vi "Select_Alternative_channel.vi"(4 "Filetype":string, 5 "All Tabulated Channels":string[](array[string]), 6 "Reading Filename":path, 7 "Start of data (bytes)":i32, 8 "Template Channel Name":string, 9 "Data string":string, 10 "Previous Channels used":string[](array[string])) -> (0 "Chosen Channel":string, 3 "Selected Index":i32)   [LabVIEW 2016]
uses:
  Results_plotter_Global.vi
panel:
  in  "Cancel Button":bool
  out "Channel Values":dbl[](graph)
  out "Channel Values":string[](array[string])
  out "Message":string
  in  "Boolean":bool
  in  "Select channel to be used":u16(ring) items=["No Suitable Channel Found", "No Suitable Channel Found, Don't Prompt again", "MyFirstName:MySecondName:Frequency (Hz)", "MyFirstName:MySecondName:Boost", "MyFirstName:MySecondName:Phase", "Port::", "L (ft)::", "Tube::", "Trans DeadL (in)::", "Pitot DeadL (in)::", "pold^2/pref^2::", "pnew^2/pref^2::", "pref^2::", "pold^2::", "pnew^2::", "User Comments::", "Pref Mean (V)::", "Pold Mean (V)::", "Pnew Mean (V)::", "Pref Timescale Estimate (s)::", "Pold Timescale Estimate (s)::", "Pnew Timescale Estimate (s)::", "Date of Measurement::", "Time Measurement Commenced::", "Seconds since 1st Jan::", "Measuring Instrument Type::", "Run Messages::", "Av Analogue Sampling Rate::", "No of Analogue Samples::", "No Of Measurement Blocks::", "Flow Measurement Time::", "Prog Post Process Mode::", "Acquisition PlugIn Used::", "Initial PlugIns Used::", "Per Block PlugIns Used::", "Raw Data Filename::", "Current:File:", "Current:File:1st Folder level", "Current:File:2nd Folder level", "Current:File:3rd Folder level", "Current:File:4th Folder level", "Current:File:Number"]
  # "#ToDo- add filter to make it easier to find channels!"
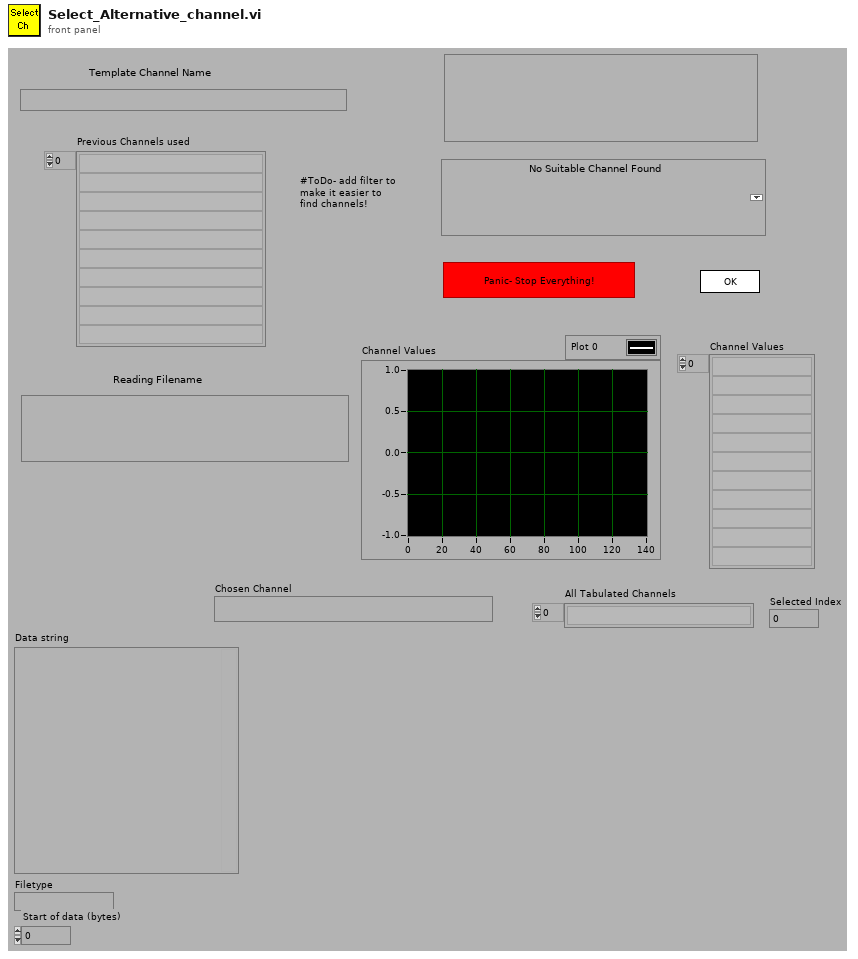
[diagram p1: front panel]
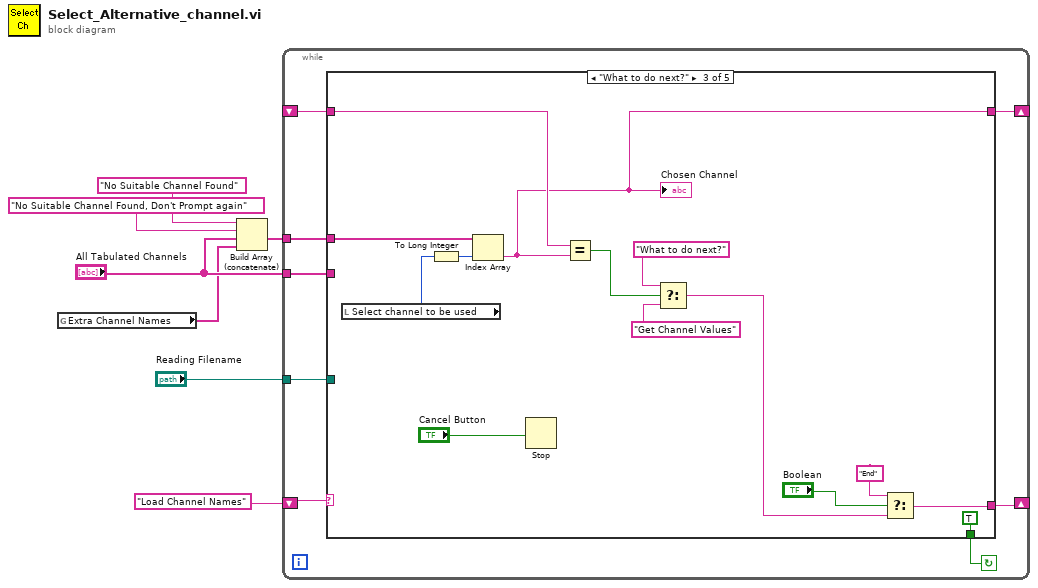
[diagram p0: block diagram]
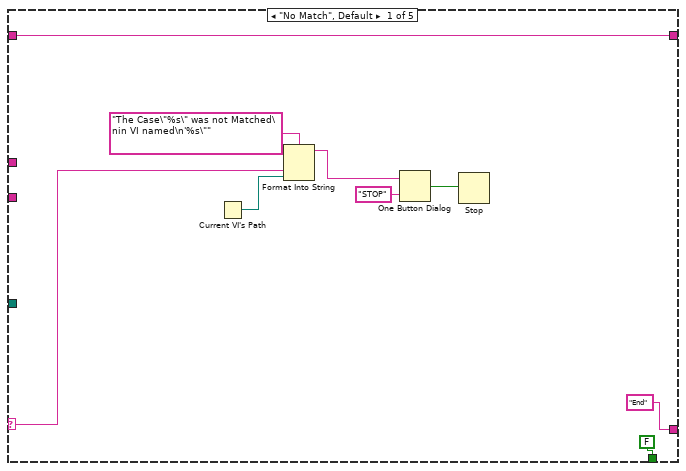
[diagram p2: hidden frame]
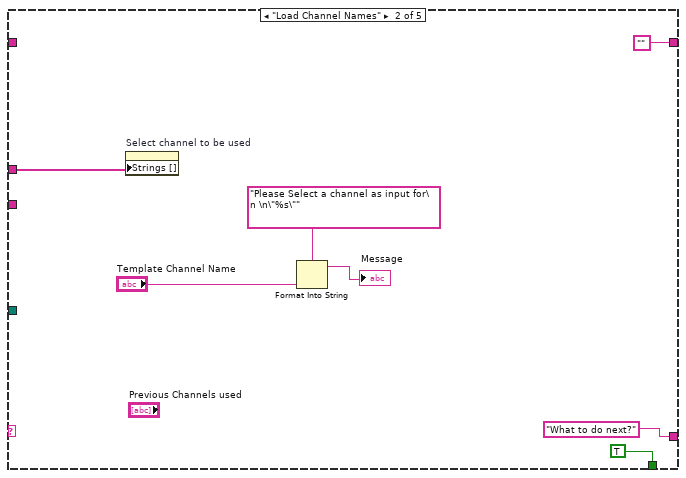
[diagram p3: hidden frame]
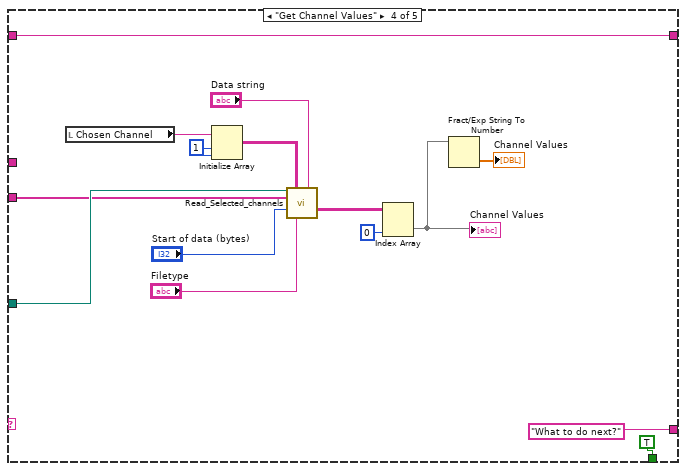
[diagram p4: hidden frame]
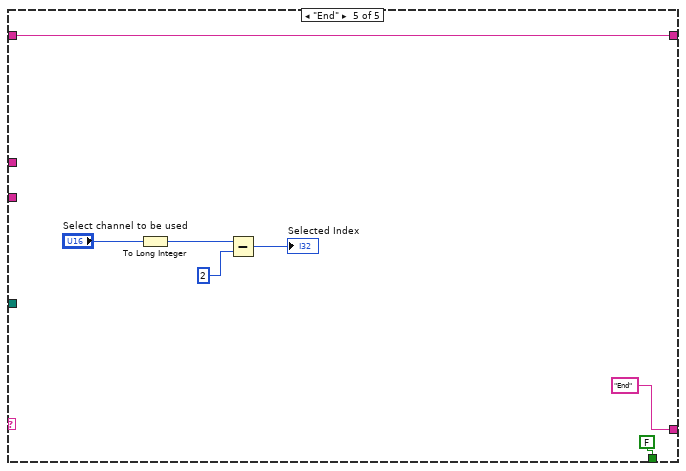
[diagram p5: hidden frame]
diagram:
  n1 = global read "Results_plotter_Global.vi" "Extra Channel Names"() -> (w1:string[])
  n2 = Build Array (concatenate)("No Suitable Channel Found" ("Input Element"), "No Suitable Channel Found, Don't Prompt again" ("Input Element"), "All Tabulated Channels", w1) -> (w5:string[])
  n3 = while {
    tunnel: w5 -> [w14]
    shift-left: "Load Channel Names" -> [w12]
    shift-right: [w13] -> _
    tunnel: "Reading Filename" -> [w11]
    tunnel: "All Tabulated Channels" -> [w10]
    shift-right: [w8] -> _
    shift-left: _ -> [w9]
    stop <- w15 continue-if-true
    n4 = case shown="\"What to do next?\"" w12 {
      selector: w12 -> [w16 _ _ _ _]
      tunnel: [FALSE TRUE TRUE TRUE FALSE] -> w15
      tunnel: w14 -> [_ w30 w40 _ _]
      tunnel: ["End" "What to do next?" w42 "What to do next?" "End"] -> w13
      tunnel: w11 -> [_ _ _ w59 _]
      tunnel: w10 -> [_ _ _ w58 _]
      tunnel: w9 -> [w17 _ w38 w47 w62]
      tunnel: [w17 "" w37 w47 w62] -> w8
      frame "No Match", Default {
        n5 = Current VI's Path() -> (path=w24:path)
        n6 = Format Into String(format string="The Case\"%s\" was not Matched\nin VI named\n'%s\"" ("Format String"), w16, w24) -> (resulting string=w21:string)  [unwired: 2 in, 1 out]
        n7 = One Button Dialog(message=w21, button name ("OK")="STOP") -> (true=w23:bool)
        n8 = Stop(stop? (T)=w23) -> ()
      }
      frame "Load Channel Names" {
        n9 = property on="Select channel to be used" class="Ring (strict)"("Strings []"=w30) -> ()  [unwired: 2 in, 2 out]
        n10 = Format Into String(format string="Please Select a channel as input for\n \n\"%s\"" ("Format String"), "Template Channel Name") -> (resulting string=→"Message":string)  [unwired: 2 in, 1 out]
      }
      frame "What to do next?" {
        n11 = local read "Select channel to be used"() -> (w45:u16)
        n12 = To Long Integer(number=w45) -> (32bit integer=w39:i32)
        n13 = Index Array(array=w40, index=w39) -> (element=w37:string)
        "Chosen Channel" <- w37
        n14 = Stop(stop? (T)="Cancel Button") -> ()
        n15 = Equal?(x=w38, y=w37) -> (x = y?=w34:bool)
        n16 = Select(t="What to do next?", s=w34, f="Get Channel Values") -> (s? t:f=w33:string)
        n17 = Select(t="End", s="Boolean", f=w33) -> (s? t:f=w42:string)
      }
      frame "Get Channel Values" {
        w56 = 1 ("dimension size")
        n18 = local read "Chosen Channel"() -> (w57:string)
        n19 = Initialize Array(w57, w56, w56) -> (w55:string[][])
        n20 = call "Read_Selected_channels.vi"("Filename"=w59, "Valid Channel Options"=w55, "Data string"="Data string", "All Channels Present"=w58, "Start of data (bytes)"="Start of data (bytes)", "Filetype"="Filetype") -> ("Output Values"=w51:string[][])  [unwired: 4 in, 5 out]
        n21 = Index Array(array=w51, index (col)=0 ("index (row)")) -> (element=w50:string[])  [unwired: 1 in]
        "Channel Values" <- w50
        n22 = Fract/Exp String To Number(string=w50) -> (number=→"Channel Values":dbl[])  [unwired: 4 out]
      }
      frame "End" {
        n23 = To Long Integer(number="Select channel to be used") -> (32bit integer=w61:i32)
        n24 = Subtract(x=w61, y=2) -> (x-y=→"Selected Index":i32)
      }
    }
  }
